vi "Build.vi"(1 "timeout (ms)":i32=30000, 2 "mode":T1=enum."N/A", 3 "Deadline in":T2={"mode"=enum."Relative", "deadline (ms)"=30000}) -> (0 "Deadline out":T2={"mode"=enum."Relative", "deadline (ms)"=30000})   [LabVIEW 2020, in "NI_Deadline.lvlib"]
uses:
  <vilib>/Utility/Deadline/NI_Deadline.lvlib
  <vilib>/Utility/Deadline/Deadline.ctl
  <vilib>/Utility/Deadline/Mode.ctl
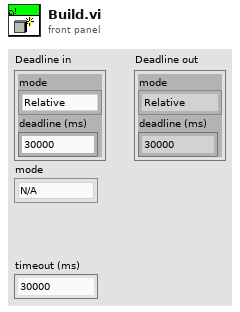
[diagram p1: front panel]
types:
  T1 = typedef "NI_Deadline.lvlib/Mode.ctl" = enum16{"Relative", "Use deadline", "Wait forever", "Nonblocking", "N/A"}
  T2 = typedef "NI_Deadline.lvlib/Deadline.ctl" = cluster{"mode":T1, "deadline (ms)":u32}
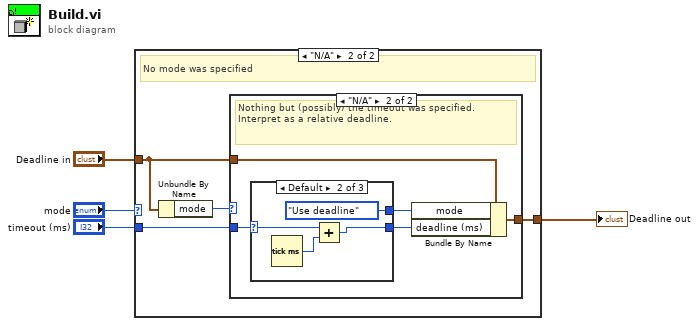
[diagram p0: block diagram]
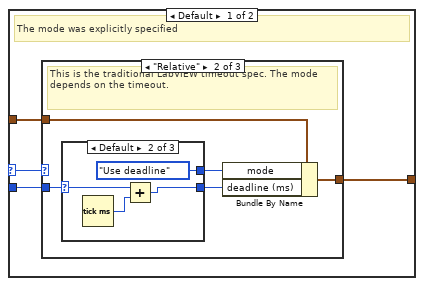
[diagram p2: hidden frame]
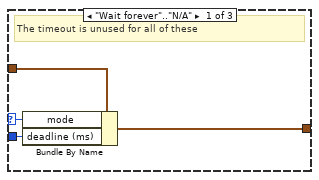
[diagram p3: hidden frame]
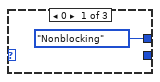
[diagram p4: hidden frame]
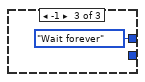
[diagram p5: hidden frame]
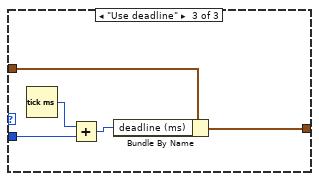
[diagram p6: hidden frame]
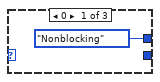
[diagram p8: hidden frame]
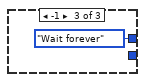
[diagram p9: hidden frame]
diagram:
  n1 = case shown="\"N/A\"" "mode" {
    selector: "mode" -> [w8 _]
    tunnel: "Deadline in" -> [w5 w31]
    tunnel: [w6 w29] -> w2
    tunnel: "timeout (ms)" -> [w7 w30]
    frame Default {
      # "The mode was explicitly specified"
      n2 = case shown="\"Relative\"" w8 {
        selector: w8 -> [w10 _ _]
        tunnel: w7 -> [w9 w17 w26]
        tunnel: [w11 w16 w27] -> w6
        tunnel: w5 -> [w12 w13 w28]
        frame "Wait forever".."N/A" {
          # "The timeout is unused for all of these"
          n3 = Bundle By Name(cluster=w12, "mode"=w10, "deadline (ms)"=w9) -> (w11:T2)
        }
        frame "Relative" {
          # "This is the traditional LabVIEW timeout spec. The mode depends on the timeout."
          n4 = case shown="Default" w17 {
            selector: w17 -> [_ w21 _]
            tunnel: [Mode."Nonblocking" ("mode") Mode."Use deadline" ("mode") Mode."Wait forever" ("mode")] -> w15
            tunnel: [_ w19 _] -> w14
            frame 0 {
            }
            frame Default {
              n5 = Tick Count (ms)() -> (millisecond timer value=w20:u32)
              n6 = Add(x=w21, y=w20) -> (x+y=w19:u32)
            }
            frame -1 {
            }
          }
          n7 = Bundle By Name(cluster=w13, "mode"=w15, "deadline (ms)"=w14) -> (w16:T2)
        }
        frame "Use deadline" {
          n8 = Tick Count (ms)() -> (millisecond timer value=w25:u32)
          n9 = Add(x=w25, y=w26) -> (x+y=w24:u32)
          n10 = Bundle By Name(cluster=w28, "deadline (ms)"=w24) -> (w27:T2)
        }
      }
    }
    frame "N/A" {
      # "No mode was specified"
      n11 = Unbundle By Name(w31) -> ("mode"=w32:T1)
      n12 = case shown="\"N/A\"" w32 {
        tunnel: w31 -> [w33 w35]
        tunnel: w30 -> [_ w36]
        tunnel: [w33 w34] -> w29
        frame Default {
          # "The deadline has been initialized but the mode hasn't; use the deadline verbatim"
        }
        frame "N/A" {
          # "Nothing but (possibly) the timeout was specified. Interpret as a relative deadline."
          n13 = case shown="Default" w36 {
            selector: w36 -> [_ w42 _]
            tunnel: [Mode."Nonblocking" ("mode") Mode."Use deadline" ("mode") Mode."Wait forever" ("mode")] -> w38
            tunnel: [_ w40 _] -> w37
            frame 0 {
            }
            frame Default {
              n14 = Tick Count (ms)() -> (millisecond timer value=w41:u32)
              n15 = Add(x=w42, y=w41) -> (x+y=w40:u32)
            }
            frame -1 {
            }
          }
          n16 = Bundle By Name(cluster=w35, "mode"=w38, "deadline (ms)"=w37) -> (w34:T2)
        }
      }
    }
  }
  "Deadline out" <- w2
